vi "Keithley4200 Plot list sweep.vi"() -> ()   [LabVIEW 2013]
uses:
  <vilib>/Instr/_visa.llb/VISA Event Mechanism.ctl
  <vilib>/Instr/_visa.llb/Select Event Type.ctl
panel:
  out "Resistance (Ohm)":dbl
  out "Current (A)    Voltage (V)":dbl[][](array[numeric]) caption="appended array"
  out "XY Graph":cluster{dbl[], dbl[]}(graph)
  out "error out":errorcluster={"status"=TRUE, "code"=-1073807346, "source"="VISA Open in 4200MOSFETexample1.vi"}
  # "4-Point Measurement\nSMU1 = current source\nSMU2 = COM"
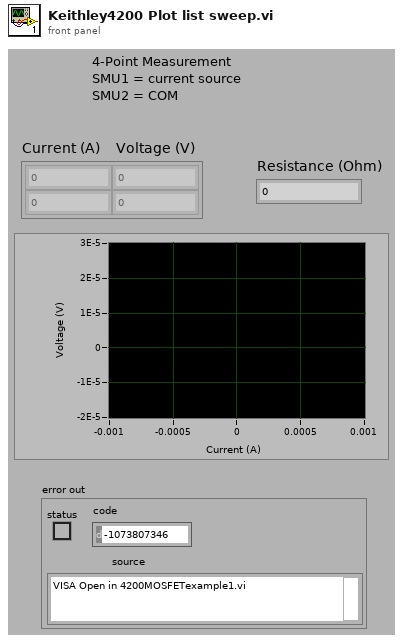
[diagram p1: front panel]
types:
  T1 = typedef "Select Event Type.ctl" = u32
  T2 = typedef "VISA Event Mechanism.ctl" = u16
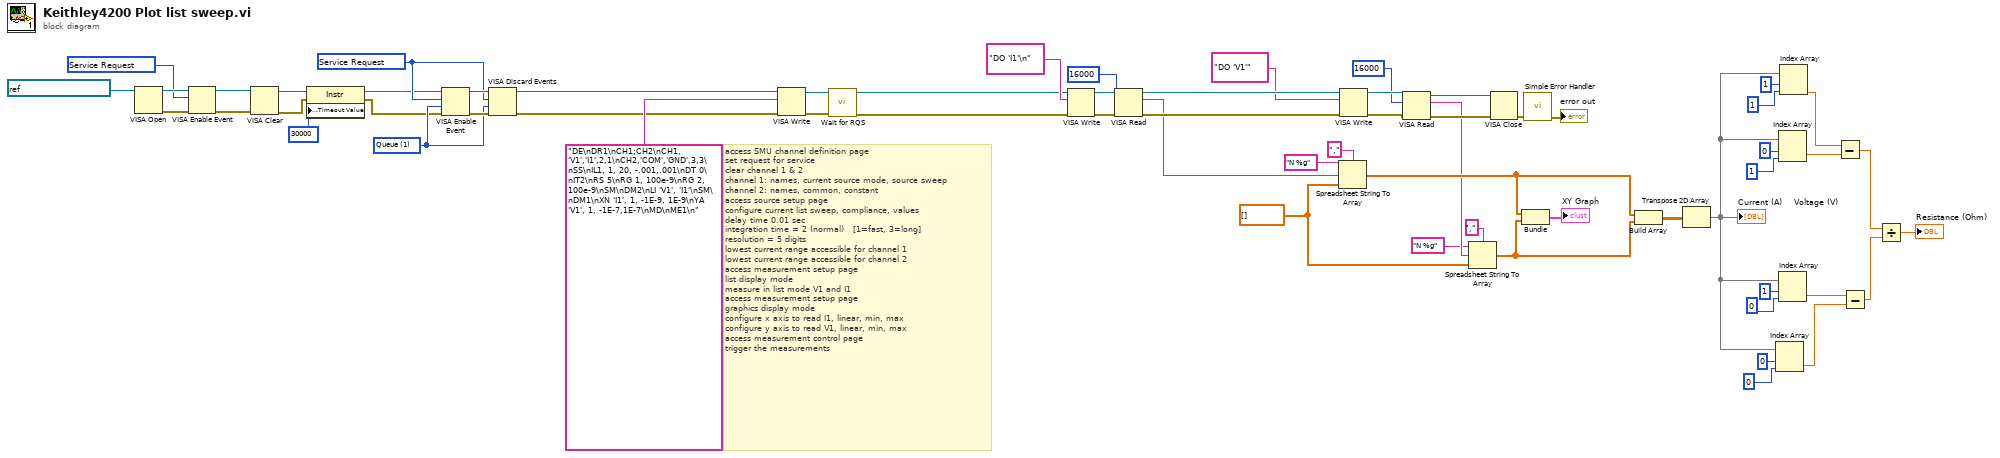
[diagram p0: block diagram]
diagram:
  w10 = T1 1073684491 items=["Service Request"=1073684491, "Trigger"=3221168138, "Clear"=1073684493, "VXI Signal"=1073684512, "VXI/VME Interrupt"=3221168161, "VXI/VME Sysfail"=1073684509, "VXI/VME Sysreset"=1073684510, "GPIB CIC"=1073684498, "GPIB Talk"=1073684499, "GPIB Listen"=1073684500, "PXI Interrupt"=1073684514, "Serial Break"=1073684515, "Serial TermChar"=1073684516, "Serial CTS"=1073684521, "Serial DSR"=1073684522, "Serial DCD"=1073684524, "Serial RI"=1073684526, "Serial Character"=1073684533, "USB Interrupt"=1073684535, "All Enabled"=1073709055] ("Event Type")
  w19 = T2 1 items=["Queue"=1] ("Mechanism Type")
  w20 = T1 1073684491 items=["Service Request"=1073684491, "Trigger"=3221168138, "Clear"=1073684493, "VXI Signal"=1073684512, "VXI/VME Interrupt"=3221168161, "VXI/VME Sysfail"=1073684509, "VXI/VME Sysreset"=1073684510, "GPIB CIC"=1073684498, "GPIB Talk"=1073684499, "GPIB Listen"=1073684500, "PXI Interrupt"=1073684514, "Serial Break"=1073684515, "Serial TermChar"=1073684516, "Serial CTS"=1073684521, "Serial DSR"=1073684522, "Serial DCD"=1073684524, "Serial RI"=1073684526, "Serial Character"=1073684533, "USB Interrupt"=1073684535, "All Enabled"=1073709055] ("Event Type")
  w49 = dbl[] []
  # "access SMU channel definition page\nset request for service\nclear channel 1 & 2\nchannel 1: names, current source mode, source sweep\nchannel 2: names, common, constant\naccess source setup page\nconfigure current list sweep, compliance, values\ndelay time 0.01 sec\nintegration time = 2 (normal)   [1=fast, 3=long]\nresolution = 5 digits\nlowest current range accessible for channel 1\nlowest current range accessible for channel 2\naccess measurement setup page\nlist display mode\nmeasure in list mode V1 and I1\naccess measurement setup page\ngraphics display mode\nconfigure x axis to read I1, linear, min, max\nconfigure y axis to read V1, linear, min, max\naccess measurement control page\ntrigger the measurements"
  n1 = VISA Open(VISA resource name=refnum<visa-resource-name> "GPIB0::17::INSTR") -> (VISA resource name=w13:refnum<visa-resource-name>, error out=w14:errorcluster)  [unwired: 1 in, 3 out]
  n2 = VISA Enable Event(8:w14, 10:w10, 11:w13) -> (0:w11:errorcluster, 3:w12:refnum<visa-resource-name>)  [unwired: 1 out]
  n3 = VISA Clear(VISA resource name=w12, error in (no error)=w11) -> (VISA resource name out=w18:refnum<visa-resource-name>, error out=w17:errorcluster)
  n4 = property class="Instr"(reference=w18, error in=w17, "General Settings:Timeout Value"=u32 30000) -> (reference out=w16:refnum<visa-resource-name>, error out=w15:errorcluster)
  n5 = VISA Enable Event(8:w15, 9:w19, 10:w20, 11:w16) -> (0:w21:errorcluster, 3:w22:refnum<visa-resource-name>)
  n6 = VISA Discard Events(8:w21, 9:w19, 10:w20, 11:w22) -> (0:w5:errorcluster, 3:w6:refnum<visa-resource-name>)
  n7 = VISA Write(VISA resource name=w6, write buffer="DE\nDR1\nCH1;CH2\nCH1, 'V1','I1',2,1\nCH2,'COM','GND',3,3\nSS\nIL1, 1, 20, -.001,.001\nDT 0\nIT2\nRS 5\nRG 1, 100e-9\nRG 2, 100e-9\nSM\nDM2\nLI 'V1', 'I1'\nSM\nDM1\nXN 'I1', 1, -1E-9, 1E-9\nYA 'V1', 1, -1E-7,1E-7\nMD\nME1\n", error in (no error)=w5) -> (VISA resource name out=w8:refnum<visa-resource-name>, error out=w9:errorcluster)  [unwired: 1 out]
  n8 = call <vilib>:"Wait for RQS.vi"("error in (no error)"=w9, "VISA resource name"=w8) -> ("error out"=w3:errorcluster, "VISA resource name out"=w4:refnum<visa-resource-name>)  [unwired: 1 in, 7 out]
  n9 = VISA Write(VISA resource name=w4, write buffer="DO 'I1'\n", error in (no error)=w3) -> (VISA resource name out=w59:refnum<visa-resource-name>, error out=w55:errorcluster)  [unwired: 1 out]
  n10 = VISA Read(VISA resource name=w59, byte count=u32 16000, error in (no error)=w55) -> (VISA resource name out=w57:refnum<visa-resource-name>, read buffer=w42:string, error out=w53:errorcluster)  [unwired: 1 out]
  n11 = Spreadsheet String To Array(delimiter (Tab)=",", format string="N %g", spreadsheet string=w42, array type (2D Dbl)=w49) -> (array=w46:dbl[])
  n12 = VISA Write(VISA resource name=w57, write buffer="DO 'V1'", error in (no error)=w53) -> (VISA resource name out=w51:refnum<visa-resource-name>, error out=w52:errorcluster)  [unwired: 1 out]
  n13 = VISA Read(VISA resource name=w51, byte count=u32 16000, error in (no error)=w52) -> (VISA resource name out=w63:refnum<visa-resource-name>, read buffer=w41:string, error out=w62:errorcluster)  [unwired: 1 out]
  n14 = Spreadsheet String To Array(delimiter (Tab)=",", format string="N %g", spreadsheet string=w41, array type (2D Dbl)=w49) -> (array=w45:dbl[])
  n15 = VISA Close(VISA resource name=w63, error in (no error)=w62) -> (error out=w61:errorcluster)
  n16 = Bundle(w46, w45) -> (→"XY Graph":cluster{dbl[], dbl[]})  [unwired: 1 in]
  n17 = call <vilib>:"Simple Error Handler.vi"("error in (no error)"=w61) -> ("error out"=→"error out":errorcluster)  [unwired: 4 in, 4 out]
  n18 = Build Array(w46, w45) -> (w43:dbl[][])
  n19 = Transpose 2D Array(2D array=w43) -> (transposed array=w27:dbl[][])
  "Current (A)    Voltage (V)" <- w27
  n20 = Index Array(array=w27, index (row)=0, index (col)=0 ("index (row)")) -> (element=w31:dbl)
  n21 = Index Array(array=w27, index (row)=0, index (col)=1 ("index (row)")) -> (element=w28:dbl)
  n22 = Index Array(array=w27, index (row)=1, index (col)=0 ("index (row)")) -> (element=w32:dbl)
  n23 = Index Array(array=w27, index (row)=1, index (col)=1 ("index (row)")) -> (element=w29:dbl)
  n24 = Subtract(x=w29, y=w28) -> (x-y=w25:dbl)
  n25 = Subtract(x=w32, y=w31) -> (x-y=w26:dbl)
  n26 = Divide(x=w25, y=w26) -> (x/y=→"Resistance (Ohm)":dbl)
